vi "SI657.vi"(0 "SI657.lvclass":refnum<class "SI657.lvclass">, 1 "PG Factor":dbl, 2 "Analog Signals from turbine":T1, 5 "error in (no error)":errorcluster) -> (12 "PG SP-Grad":dbl, 14 "SI657.lvclass out":refnum<class "SI657.lvclass">, 15 "PG SP lift-up and 4":dbl, 16 "PG eff SP":dbl, 17 "Switch Ps-Ps_d":dbl, 18 "PG target SP":dbl, 19 "error out":errorcluster)   [LabVIEW 2022 SP3, in "SI657.lvclass"]
uses:
  SI657.lvclass
  SI657.lvclass/SI657.ctl
panel:
  # "SI657"
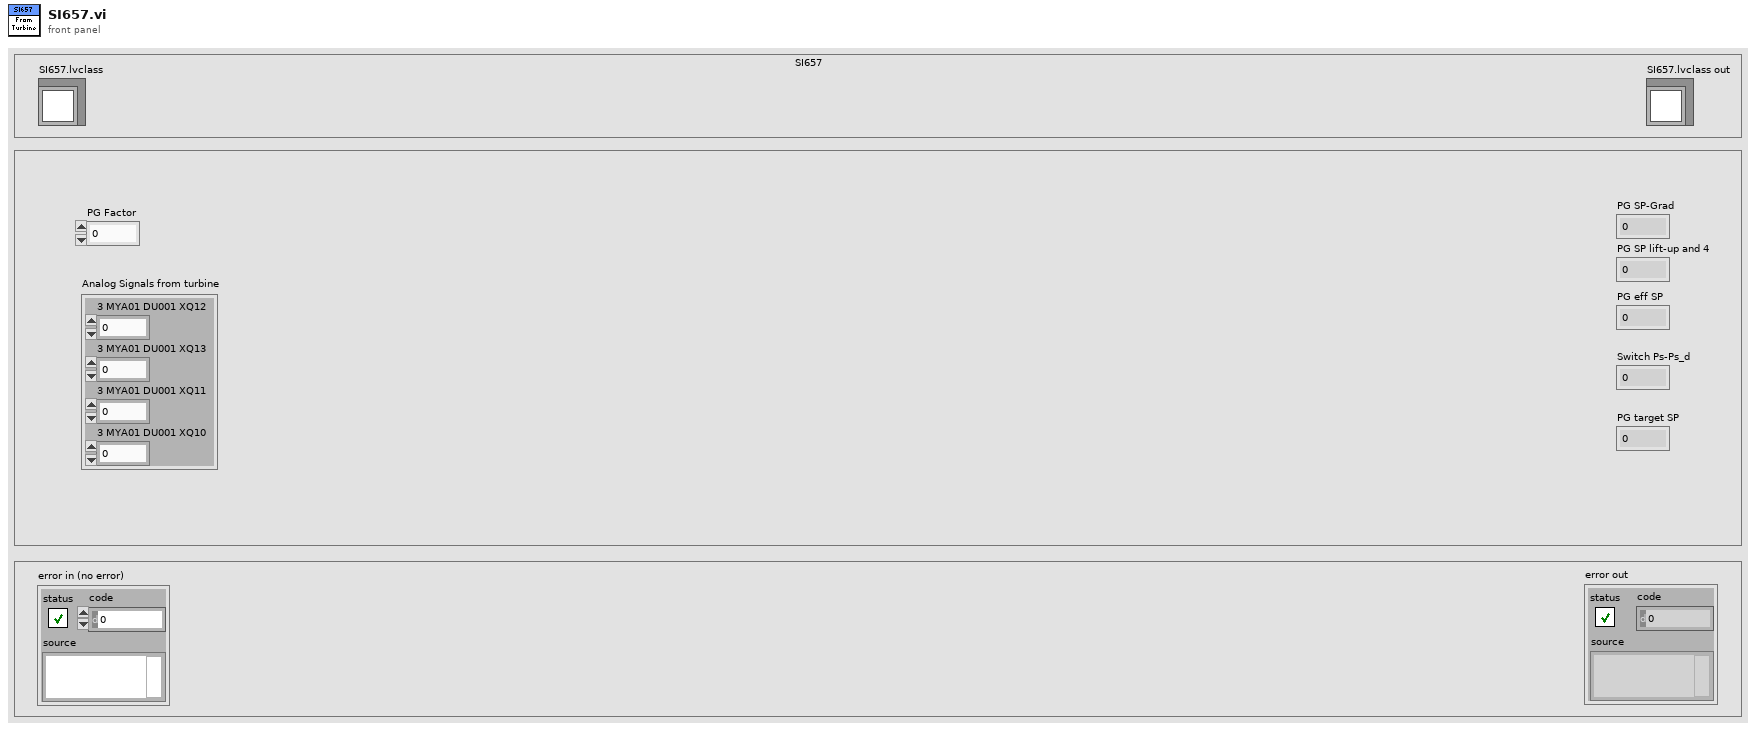
[diagram p1: front panel]
types:
  T1 = cluster{"3 MYA01 DU001 XQ12":dbl, "3 MYA01 DU001 XQ13":dbl, "3 MYA01 DU001 XQ11":dbl, "3 MYA01 DU001 XQ10":dbl}
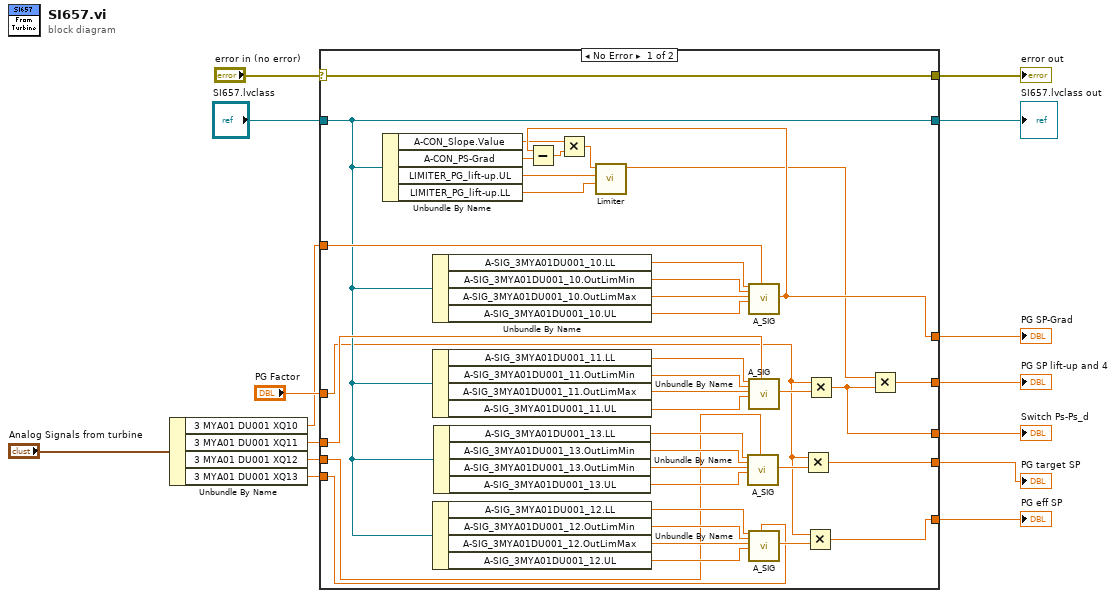
[diagram p0: block diagram]
diagram:
  n1 = Unbundle By Name("Analog Signals from turbine") -> ("3 MYA01 DU001 XQ10"=w1:dbl, "3 MYA01 DU001 XQ11"=w2:dbl, "3 MYA01 DU001 XQ12"=w4:dbl, "3 MYA01 DU001 XQ13"=w3:dbl)
  n2 = case shown="No Error" "error in (no error)" {
    selector: "error in (no error)" -> [w53 w54]
    tunnel: [w53 w54] -> w14
    tunnel: [w42 _] -> w13
    tunnel: [w41 _] -> w12
    tunnel: [w18 _] -> w11
    tunnel: [w45 _] -> w10
    tunnel: [w40 _] -> w9
    tunnel: "SI657.lvclass" -> [w19 _]
    tunnel: "PG Factor" -> [w16 _]
    tunnel: [w19 _] -> w6
    tunnel: w4 -> [w21 _]
    tunnel: w3 -> [w20 _]
    tunnel: w2 -> [w51 _]
    tunnel: w1 -> [w50 _]
    frame No Error {
      n3 = Unbundle By Name(w19) -> ("A-CON_Slope.Value"=w44:dbl, "A-CON_PS-Grad"=w46:dbl, "LIMITER_PG_lift-up.UL"=w39:dbl, "LIMITER_PG_lift-up.LL"=w38:dbl)
      n4 = Unbundle By Name(w19) -> ("A-SIG_3MYA01DU001_10.LL"=w25:dbl, "A-SIG_3MYA01DU001_10.OutLimMin"=w24:dbl, "A-SIG_3MYA01DU001_10.OutLimMax"=w23:dbl, "A-SIG_3MYA01DU001_10.UL"=w22:dbl)
      n5 = Unbundle By Name(w19) -> ("A-SIG_3MYA01DU001_11.LL"=w29:dbl, "A-SIG_3MYA01DU001_11.OutLimMin"=w28:dbl, "A-SIG_3MYA01DU001_11.OutLimMax"=w27:dbl, "A-SIG_3MYA01DU001_11.UL"=w26:dbl)
      n6 = Unbundle By Name(w19) -> ("A-SIG_3MYA01DU001_12.LL"=w37:dbl, "A-SIG_3MYA01DU001_12.OutLimMin"=w36:dbl, "A-SIG_3MYA01DU001_12.OutLimMax"=w35:dbl, "A-SIG_3MYA01DU001_12.UL"=w34:dbl)
      n7 = Unbundle By Name(w19) -> ("A-SIG_3MYA01DU001_13.LL"=w33:dbl, "A-SIG_3MYA01DU001_13.OutLimMin"=w32:dbl, "A-SIG_3MYA01DU001_13.OutLimMin"=w31:dbl, "A-SIG_3MYA01DU001_13.UL"=w30:dbl)
      n8 = call "A_SIG.vi"("LL"=w33, "OutLimMin"=w32, "OutLimMax"=w31, "UL"=w30, "Input"=w21) -> ("A_SIG_out"=w48:dbl)  [unwired: 13 in, 1 out]
      n9 = call "A_SIG.vi"("LL"=w25, "OutLimMin"=w24, "OutLimMax"=w23, "UL"=w22, "Input"=w50) -> ("A_SIG_out"=w45:dbl)  [unwired: 13 in, 1 out]
      n10 = Subtract(x=w45, y=w46) -> (x-y=w52:dbl)
      n11 = Multiply(x=w44, y=w52) -> (x*y=w43:dbl)
      n12 = call "Limiter.vi"("LIMITER_PG_lift-up.LL"=w38, "LIMITER_PG_lift-up.UL in"=w39, "input"=w43) -> ("LIMITER_PG_lift-up.UL out"=w17:dbl)  [unwired: 5 in, 3 out]
      n13 = call "A_SIG.vi"("LL"=w29, "OutLimMin"=w28, "OutLimMax"=w27, "UL"=w26, "Input"=w51) -> ("A_SIG_out"=w47:dbl)  [unwired: 13 in, 1 out]
      n14 = call "A_SIG.vi"("LL"=w37, "OutLimMin"=w36, "OutLimMax"=w35, "UL"=w34, "Input"=w20) -> ("A_SIG_out"=w49:dbl)  [unwired: 13 in, 1 out]
      n15 = Multiply(x=w16, y=w48) -> (x*y=w41:dbl)
      n16 = Multiply(x=w16, y=w49) -> (x*y=w42:dbl)
      n17 = Multiply(x=w16, y=w47) -> (x*y=w18:dbl)
      n18 = Multiply(x=w17, y=w18) -> (x*y=w40:dbl)
    }
    frame Error {
    }
  }
  "error out" <- w14
  "SI657.lvclass out" <- w6
  "PG eff SP" <- w13
  "PG target SP" <- w12
  "Switch Ps-Ps_d" <- w11
  "PG SP-Grad" <- w10
  "PG SP lift-up and 4" <- w9
